vi "Write Raw.vi"(8 "error in (no error)":errorcluster, 10 "Path":path, 11 "ImageHandler in":refnum<class "ImageHandler.lvclass">) -> (0 "error out":errorcluster, 3 "ImageHandler out":refnum<class "ImageHandler.lvclass">)   [LabVIEW 2022 SP3, in "ImageHandler.lvlib" / "ImageHandler.lvclass"]
uses:
  ImageHandler.lvclass
  ImageHandler.lvclass/ImageHandler.ctl
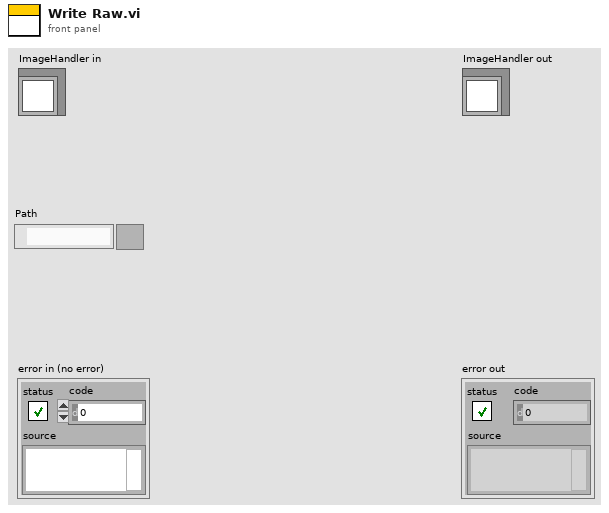
[diagram p1: front panel]
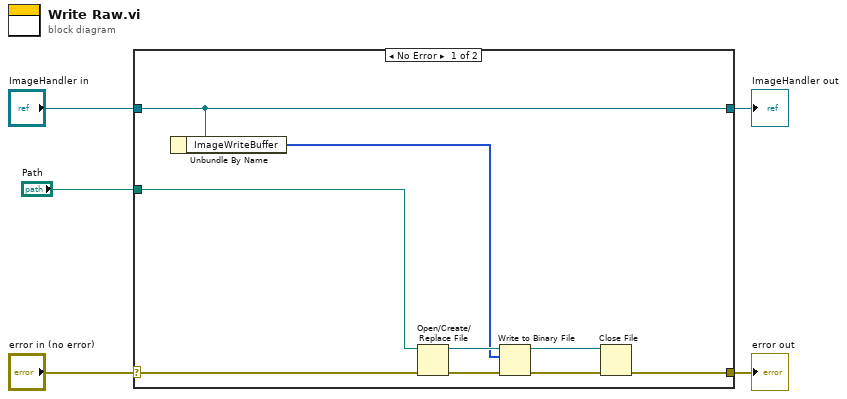
[diagram p0: block diagram]
diagram:
  n1 = case shown="No Error" "error in (no error)" {
    selector: "error in (no error)" -> [w14 w16]
    tunnel: [w10 w16] -> w4
    tunnel: [w13 w15] -> w2
    tunnel: "ImageHandler in" -> [w13 w15]
    tunnel: "Path" -> [w8 _]
    frame No Error {
      n2 = Unbundle By Name(w13) -> ("ImageWriteBuffer"=w6:u16[])
      n3 = Open/Create/Replace File(file path (use dialog)=w8, error in=w14) -> (refnum out=w9:refnum<file>, error out=w12:errorcluster)  [unwired: 4 in, 1 out]
      n4 = Write to Binary File(file (use dialog)=w9, data=w6, error in=w12) -> (refnum out=w7:refnum<file>, error out=w11:errorcluster)  [unwired: 3 in, 1 out]
      n5 = Close File(refnum=w7, error in=w11) -> (error out=w10:errorcluster)  [unwired: 1 out]
    }
    frame Error {
    }
  }
  "error out" <- w4
  "ImageHandler out" <- w2
